vi "Winch State Transition Example.vi"() -> ()   [LabVIEW 2017]
uses:
  Global State Variables.vi
panel:
  in  "stop":bool
  in  "State Selector Methods":enum32{"using one button", "using two buttons"}(tab)
  in  "single buton selector":bool
  in  "right button\nselector":bool
  in  "left button \nselector":bool
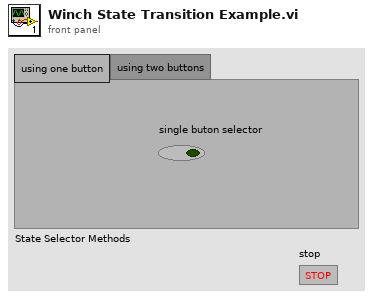
[diagram p1: front panel]
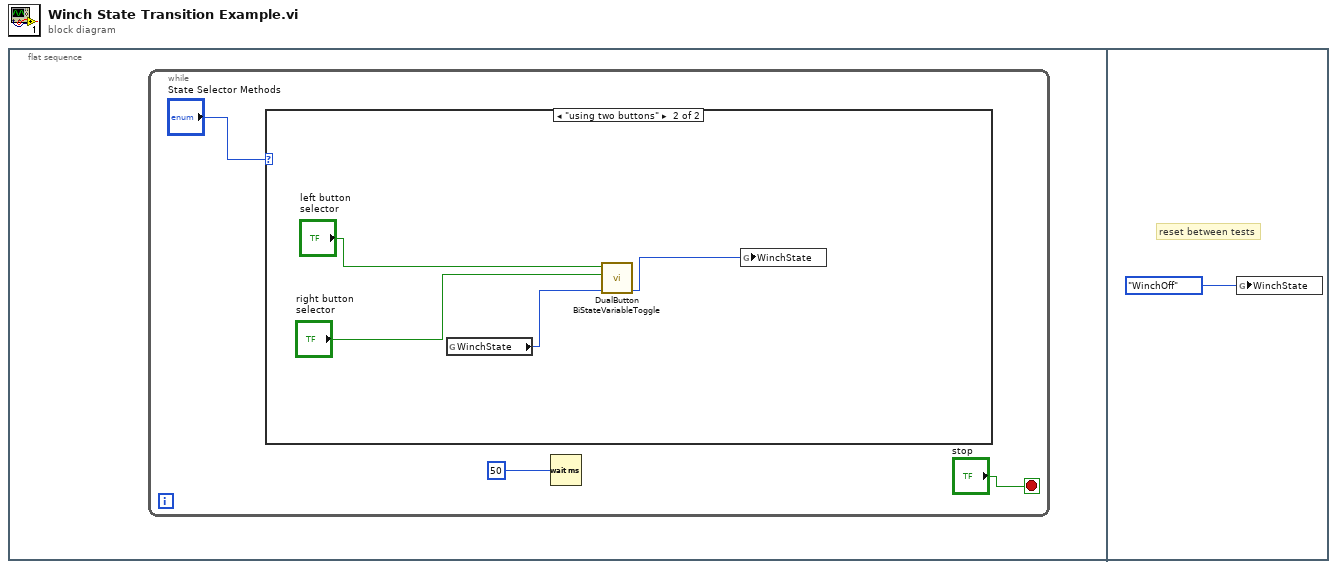
[diagram p0: block diagram]
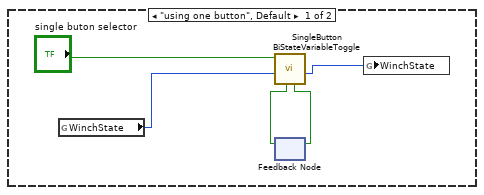
[diagram p2: hidden frame]
diagram:
  n1 = flat-sequence {
    frame #0 {
      n2 = while {
        stop <- "stop" stop-if-true
        n3 = case shown="\"using two buttons\"" "State Selector Methods" {
          frame "using one button", Default {
            n4 = global read "Global State Variables.vi" "WinchState"() -> (w4:enum16{"WinchOff", "WinchClimb", "WinchHold"})
            n5 = feedback #1() -> (w6:bool)  [unwired: 1 in]
            n6 = call "SingleButton BiStateVariableToggle.vi"("AlreadySwitched?"=w6, "PreviousState"=w4, "Button"="single buton selector") -> ("NewState"=w5:u16, "StillSwitched?"=w7:bool)  [unwired: 7 in]
            n7 = feedback-in #1(w7) -> ()
            n8 = global write "Global State Variables.vi" "WinchState"(w5) -> ()
          }
          frame "using two buttons" {
            n9 = global read "Global State Variables.vi" "WinchState"() -> (w12:enum16{"WinchOff", "WinchClimb", "WinchHold"})
            n10 = call "DualButton BiStateVariableToggle.vi"("PreviousState"=w12, "ButtonToSelect\nSecondState"="right button\nselector", "ButtonToSelect\nFirstState"="left button \nselector") -> ("NewState"=w11:u16)  [unwired: 8 in]
            n11 = global write "Global State Variables.vi" "WinchState"(w11) -> ()
          }
        }
        n12 = Wait (ms)(milliseconds to wait=u32 50) -> ()  [unwired: 1 out]
      }
    }
    frame #1 {
      # "reset between tests"
      n13 = global write "Global State Variables.vi" "WinchState"(enum16{"WinchOff", "WinchClimb", "WinchHold"}."WinchOff" ("WinchState")) -> ()
    }
  }
